vi "Bodies_GetCoM.vi"(8 "error in (no error)":errorcluster, 11 "Bodies in":refnum<class "Bodies.lvclass">) -> (0 "error out":errorcluster, 2 "CoM":T1[](array[typedef]), 3 "Bodies out":refnum<class "Bodies.lvclass">)   [LabVIEW 2015, in "Bodies.lvclass"]
uses:
  Bodies.lvclass
  PointOnBody.ctl
  Bodies.lvclass/Bodies.ctl
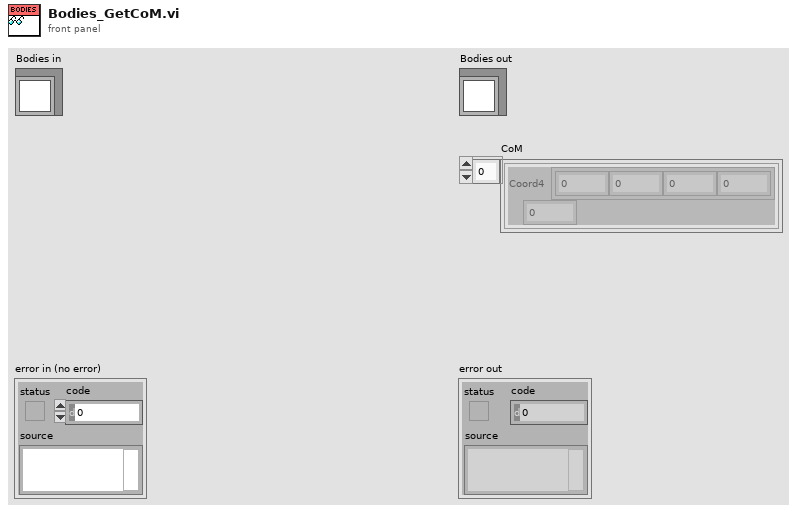
[diagram p1: front panel]
types:
  T1 = typedef "Bodies.lvclass/PointOnBody.ctl" = cluster{"Coord4":dbl[], "ID":i32}
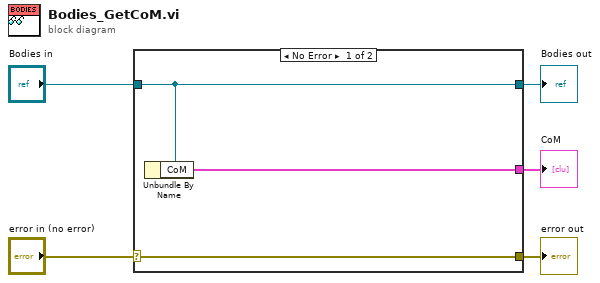
[diagram p0: block diagram]
diagram:
  n1 = case shown="No Error" "error in (no error)" {
    selector: "error in (no error)" -> [w8 w9]
    tunnel: [w8 w9] -> w4
    tunnel: [w7 w10] -> w2
    tunnel: "Bodies in" -> [w7 w10]
    tunnel: [w6 _] -> w1
    frame No Error {
      n2 = Unbundle By Name(w7) -> ("CoM"=w6:T1[])
    }
    frame Error {
    }
  }
  "error out" <- w4
  "Bodies out" <- w2
  "CoM" <- w1
